vi "RingGetcam.VI"() -> ()   [LabVIEW 2014]
panel:
  in  "gain":bool
  in  "is FFT":bool
  out "FIFO overflow":bool
  in  "RingBufDepth":u32=100
  out "Signalverlaufgraph":u16[](graph)=[1244, 50394, 4112, 1253, 7937, 7970, 8022, 8007, 8036, 8064, 8081, 8047, 8038, 8131, 8189, 8160, 8237, 8217, 8253, 8234, 8286, 8282, 8333, 8330, 8377, 8354, 8432, 8412, 8472, 8454, 8502, 8506, 8551, 8555, 8618, 8587, 8654, 8622, 8678, 8676, 8705, 8728, 8760, 8721, 8806, 8782, 8832, 8816, 8851, 8867, 8922, 8915, 8965, 8956, 9002, 9006, 9029, 9038, 9114, 9050, 9101, 9142, 9164, 9171, 9207, 9200, 9261, 9214, 9288, 9285, 9307, 9310, 9364, 9322, 9368, 9404, 9444, 9436, 9485, 9469, 9497, 9508, 9551, 9587, 9619, 9562, 9655, 9637, 9680, 9710, 9733, 9765, 9805, 9794, 9828, 9847, 9877, 9892, 9929, 9953, 9984, 9976, 9964, 9951, 10046, 10054, 10122, 10146, 10138, 10167, 10220, 10223, 10221, 10209, 10262, 10275, 10311, 10336, 10323, 10329, 10396, 10389, 10431, 10441, 10499, 10494, 10530, 10518, 10556, 10581, 10574, 10588, 10671, 10647, 10718, 10692, 10736, 10737, 10788, 10775, 10817, 10833, 10901, 10910, 10918, 10969, 10979, 10881, 10950, 11009, 11047, 11098, 11107, 11147, 11163, 11162, 11227, 11210, 11262, 11276, 11309, 11281, 11376, 11389, 11416, 11363, 11442, 11440, 11474, 11467, 11544, 11546, 11578, 11588, 11602, 11640, 11674, 11702, 11752, 11734, 11773, 11843, 11822, 11884, 11908, 11894, 11970, 11945, 11982, 11998, 12097, 12075, 12138, 12095, 12193, 12189, 12212, 12229, 12270, 12291, 12316, 12311, 12403, 12336, 12398, 12436, 12438, 12466, 12529, 12485, 12567, 12474, 12519, 12605, 12658, 12644, 12686, 12689, 12758, 12769, 12800, 12781, 12848, 12835, 12800, 12899, 12934, 12922, 13024, 13029, 13054, 13029, 13052, 13056, 13115, 13124, 13177, 13229, 13227, 13212, 13273, 13273, 13364, 13298, 13388, 13369, 13398, 13353, 13433, 13426, 13527, 13481, 13577, 13517, 13573, 13564, 13572, 13572, 13630, 13597, 13724, 13640, 13703, 13749, 13749, 13746, 13754, 13800, 13805, 13805, 13882, 13865, 13820, 13884, 13937, 13915, 13930, 13952, 13982, 14022, 13992, 13984, 14010, 14082, 14053, 14123, 14116, 14130, 14144, 14159, 14198, 14243, 14153, 14275, 14233, 14252, 14251, 14226, 14320, 14319, 14348, 14346, 14307, 14362, 14346, 14373, 14418, 14408, 14450, 14449, 14438, 14444, 14449, 14483, 14516, 14485, 14475, 14519, 14516, 14561, 14568, 14495, 14574, 14601, 14562, 14574, 14687, 14606, 14639, 14616, 14580, 14563, 14564, 14492, 14612, 14666, 14666, 14627, 14605, 14651, 14562, 14602, 14586, 14639, 14612, 14622, 14632, 14624, 14627, 14670, 14637, 14638, 14652, 14612, 14667, 14577, 14675, 14615, 14603, 14613, 14608, 14582, 14645, 14567, 14603, 14581, 14593, 14515, 14581, 14588, 14590, 14566, 14567, 14586, 14557, 14493, 14517, 14501, 14490, 14520, 14513, 14498, 14502, 14469, 14489, 14444, 14453, 14452, 14458, 14453, 14463, 14453, 14448, 14427, 14459, 14382, 14402, 14352, 14369, 14426, 14350, 14315, 14341, 14328, 14321, 14268, 14298, 14298, 14318, 14275, 14286, 14227, 14279, 14249, 14266, 14253, 14225, 14186, 14236, 14203, 14197, 14200, 14185, 14168, 14209, 14119, 14127, 14163, 14152, 14114, 14117, 14079, 14082, 14116, 14086, 14056, 14040, 14058, 14033, 14039, 14048, 13952, 14027, 13906, 13953, 13961, 13966, 13982, 13947, 13921, 13874, 13930, 13882, 13880, 13830, 13856, 13830, 13817, 13770, 13812, 13775, 13798, 13791, 13744, 13744, 13687, 13664, 13686, 13638, 13662, 13637, 13598, 13593, 13587, 13548, 13559, 13505, 13541, 13509, 13489, 13458, 13461, 13421, 13418, 13400, 13398, 13277, 13368, 13269, 13313, 13273, 13235, 13281, 13233, 13186, 13193, 13117, 13169, 13073, 13102, 13049, 13071, 12996, 13021, 12938, 12993, 12920, 12972, 12920, 12918, 12865, 12878, 12764, 12758, 12725, 12717, 1287, 1294, 1292, 1293, 1295, 1295, 1299, 1297, 1296, 1293, 1292, 1291, 1292, 1290, 1287, 1287, 1290, 1282, 1281, 1278, 1281, 1276, 1279, 1283, 1272, 1273, 1276, 1280, 1273, 1271, 1273, 1273, 1271, 1274, 1272, 1266, 1267, 1259, 1267, 1264, 1259, 1265, 1258, 1260, 1261, 1261, 1262, 1261, 1262, 1259, 1257, 1254, 1260, 1258, 1257, 1258, 1259, 1254, 1251, 1253, 1254, 1254, 1250, 1252, 1251, 1256, 1254, 1254, 1253, 1248, 1247, 1255, 1247, 1250, 1248, 1243, 1252, 1251, 1255, 1252, 1249, 1251, 1249, 1249, 0, 0, 0, 0, 0, 0, 0, 0, 0, 0, 0, 0, 0, 0, 0, 0, 0, 0, 0, 0, 0, 0, 0, 0, 0, 0, 0, 0, 0, 0, 0, 0, 0, 0, 0, 0, 0, 0, 0, 0, 0, 0, 0, 0, 0, 0, 0, 0, 0, 0, 0, 0, 0, 0, 0, 0, 0, 0, 0, 0, 0, 0, 0, 0, 0, 0, 0, 0, 0, 0, 0, 0, 0, 0, 0, 0, 0, 0, 0, 0, 0, 0, 0, 0, 0, 0, 0, 0, 0, 0, 0, 0, 0, 0, 0, 0, 0, 0, 0, 0, 0, 0, 0, 0, 0, 0, 0, 0, 0, 0, 0, 0, 0, 0, 0, 0, 0, 0, 0, 0, 0, 0, 0, 0, 0, 0, 0, 0, 0, 0, 0, 0, 0, 0, 0, 0, 0, 0, 0, 0, 0, 0, 0, 0, 0, 0, 0, 0, 0, 0, 0, 0, 0, 0, 0, 0, 0, 0, 0, 0, 0, 0, 0, 0, 0, 0, 0, 0, 0, 0, 0, 0, 0, 0, 0, 0, 0, 0, 0, 0, 0, 0, 0, 0, 0, 0, 0, 0, 0, 0, 0, 0, 0, 0, 0, 0, 0, 0, 0, 0, 0, 0, 0, 0, 0, 0, 0, 0, 0, 0, 0, 0, 0, 0, 0, 0, 0, 0, 0, 0, 0, 0, 0, 0, 0, 0, 0, 0, 0, 0, 0, 0, 0, 0, 0, 0, 0, 0, 0, 0, 0, 0, 0, 0, 0, 0, 0, 0, 0, 0, 0, 0, 0, 0, 0, 0, 0, 0, 0, 0, 0, 0, 0, 0, 0, 0, 0, 0, 0, 0, 0, 0, 0, 0, 0, 0, 0, 0, 0, 0, 0, 0, 0, 0, 0, 0, 0, 0, 0, 0, 0, 0, 0, 0, 0, 0, 0, 0, 0, 0, 0, 0, 0, 0, 0, 0, 0, 0, 0, 0, 0, 0, 0, 0, 0, 0, 0, 0, 0, 0, 0, 0, 0, 0, 0, 0, 0, 0, 0, 0, 0, 0, 0, 0, 0, 0, 0, 0, 0, 0, 0, 0, 0, 0, 0, 0, 0, 0, 0, 0, 0, 0, 0, 0, 0, 0, 0, 0, 0, 0, 0, 0, 0, 0, 0, 0, 0, 0, 0, 0, 0, 0, 0, 0, 0, 0, 0, 0, 0, 0, 0, 0, 0, 0, 0, 0, 0, 0, 0, 0, 0, 0, 0, 0, 0, 0, 0, 0, 0, 0, 0, 0, 0, 0, 0, 0, 0, 0, 0, 0, 0, 0, 0, 0, 0, 0, 0, 0, 0, 0, 0, 0, 0, 0, 0, 0, 0, 0, 0, 0, 0, 0, 0, 0, 0, 0, 0, 0, 0, 0, 0, 0, 0, 0, 0, 0, 0, 0, 0, 0, 0, 0, 0, 0, 0, 0, 0, 0, 0, 0, 0, 0, 0, 0, 0, 0, 0, 0, 0, 0, 0, 0, 0, 0, 0, 0, 0, 0, 0, 0, 0, 0, 0, 0, 0, 0, 0, 0, 0, 0, 0, 0, 0, 0, 0, 0, 0, 0, 0, 0, 0, 0, 0, 0, 0, 0, 0, 0, 0, 0, 0, 0, 0, 0, 0, 0, 0, 0, 0, 0, 0, 0, 0, 0, 0, 0, 0, 0, 0, 0, 0, 0, 0, 0, 0, 0, 0, 0, 0, 0, 0, 0, 0, 0, 0, 0, 0, 0, 0, 0, 0, 0, 0, 0, 0, 0, 0, 0, 0, 0, 0, 0, 0, 0, 0, 0, 0, 0, 0, 0, 0, 0, 0, 0, 0, 0, 0, 0, 0, 0, 0, 0, 0, 0, 0, 0, 0, 0, 0, 0, 0, 0, 0, 0, 0, 0, 0, 0, 0, 0]
  in  "Trigger":bool
  in  "Stop":bool
  in  "ClrReads":u32=4
  in  "exposuretime":dbl=1.0 format="%.2f"
  # "Start with run"
  # "be shure to use lower stop button or ESC to quit - or thread will keep on going!"
  # "in ms"
  # "ext"
  # "int"
  # "IR"
  # "lo"
  # "hi"
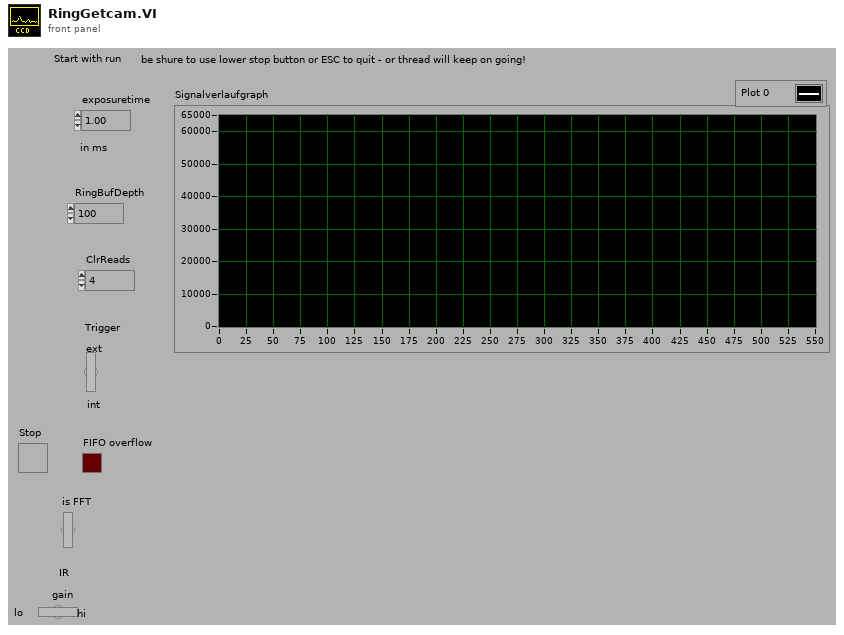
[diagram p1: front panel]
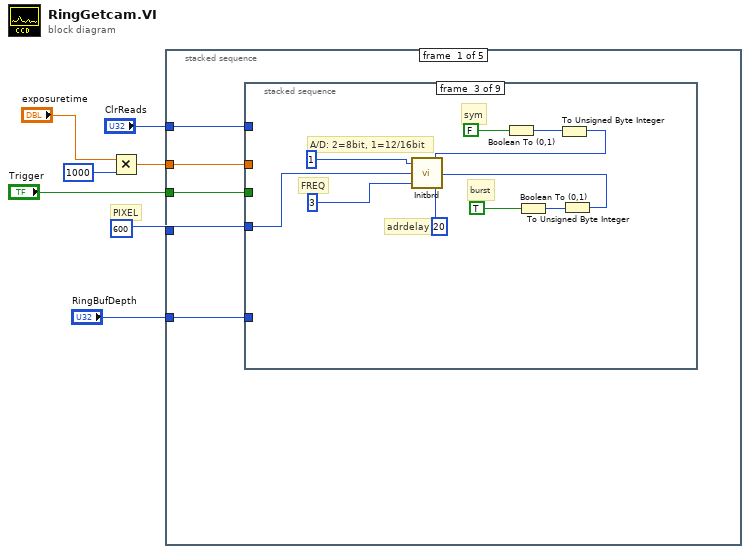
[diagram p0: block diagram]
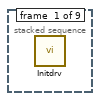
[diagram p2: hidden frame]
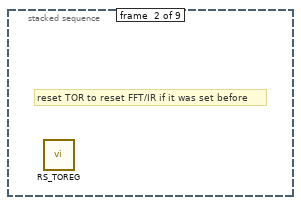
[diagram p3: hidden frame]
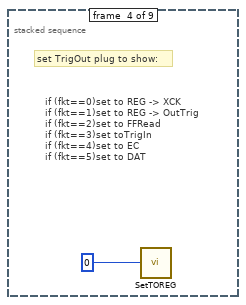
[diagram p4: hidden frame]
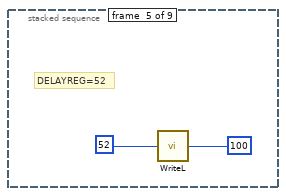
[diagram p5: hidden frame]
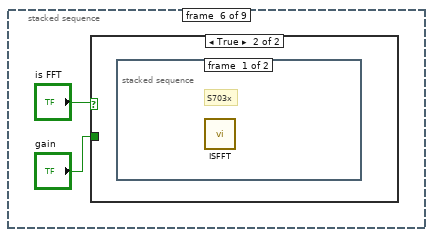
[diagram p6: hidden frame]
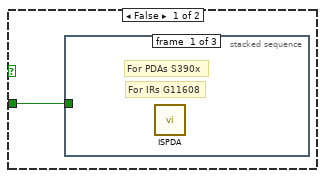
[diagram p7: hidden frame]
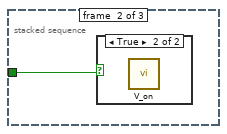
[diagram p8: hidden frame]
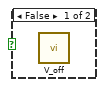
[diagram p9: hidden frame]
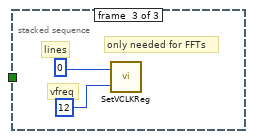
[diagram p10: hidden frame]
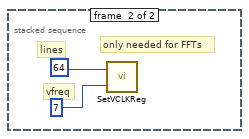
[diagram p11: hidden frame]
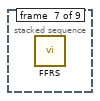
[diagram p12: hidden frame]
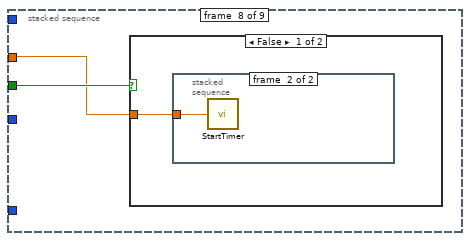
[diagram p13: hidden frame]
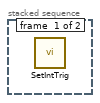
[diagram p14: hidden frame]
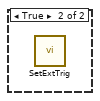
[diagram p15: hidden frame]
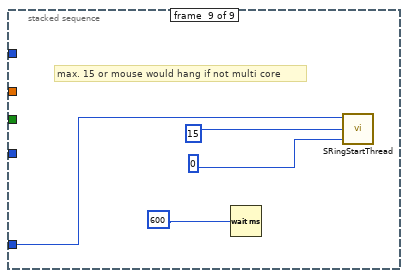
[diagram p16: hidden frame]
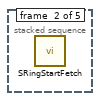
[diagram p17: hidden frame]
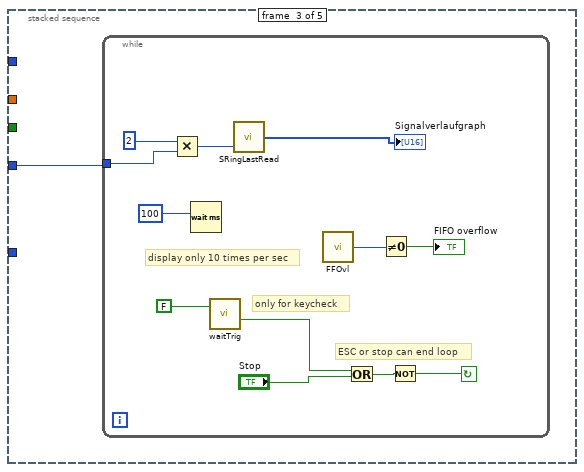
[diagram p18: hidden frame]
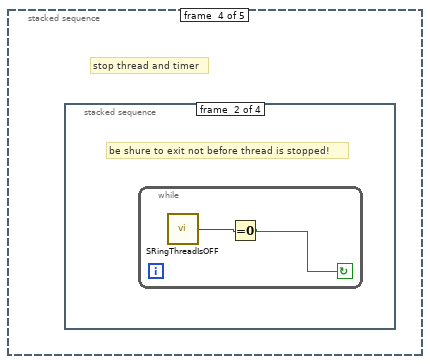
[diagram p19: hidden frame]
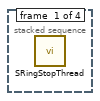
[diagram p20: hidden frame]
diagram:
  # "PIXEL"
  n1 = Multiply(x="exposuretime", y=1000) -> (x*y=w3:dbl)
  n2 = stacked-sequence {
    tunnel: w3 -> [w11 _ _ _ _]
    tunnel: u32 600 -> [w12 _ w42 _ _]
    tunnel: "ClrReads" -> [w10 _ _ _ _]
    tunnel: "Trigger" -> [w9 _ _ _ _]
    tunnel: "RingBufDepth" -> [w8 _ _ _ _]
    frame #0 {
      n3 = stacked-sequence {
        tunnel: w12 -> [_ _ w21 _ _ _ _ _ _]
        tunnel: w11 -> [_ _ _ _ _ _ _ w34 _]
        tunnel: w10 -> [_ _ _ _ _ _ _ _ _]
        tunnel: w9 -> [_ _ _ _ _ _ _ w35 _]
        tunnel: w8 -> [_ _ _ _ _ _ _ _ w38]
        frame #0 {
          n4 = call "Initdrv.vi"() -> ()  [unwired: 1 in]
        }
        frame #1 {
          # "reset TOR to reset FFT/IR if it was set before"
          n5 = call "RS_TOREG.vi"() -> ()  [unwired: 1 in]
        }
        frame #2 {
          # "adrdelay"
          # "FREQ"
          # "A/D: 2=8bit, 1=12/16bit"
          # "burst"
          # "sym"
          n6 = Boolean To (0,1)(Boolean=FALSE) -> (0, 1=w15:i16)
          n7 = Boolean To (0,1)(Boolean=TRUE) -> (0, 1=w14:i16)
          n8 = To Unsigned Byte Integer(number=w15) -> (unsigned 8bit integer=w16:u8)
          n9 = To Unsigned Byte Integer(number=w14) -> (unsigned 8bit integer=w13:u8)
          n10 = call "Initbrd.vi"("AdrDelay"=u32 20, "burst"=w13, "sym"=w16, "waits"=u32 3, "pixel"=w21, "flag816"=u32 1) -> ()
        }
        frame #3 {
          # "set TrigOut plug to show:"
          # "if (fkt==0)set to REG -> XCK\nif (fkt==1)set to REG -> OutTrig\nif (fkt==2)set to FFRead\nif (fkt==3)set toTrigIn\nif (fkt==4)set to EC\nif (fkt==5)set to DAT"
          n11 = call "SetTOREG.vi"("fkt"=u8 0) -> ()
        }
        frame #4 {
          # "DELAYREG=52"
          n12 = call "WriteL.vi"("val"=u32 100, "offset"=u32 52) -> ()
        }
        frame #5 {
          n13 = case shown="True" "is FFT" {
            tunnel: "gain" -> [w28 _]
            frame False {
              n14 = stacked-sequence {
                tunnel: w28 -> [_ w29 _]
                frame #0 {
                  # "For IRs G11608"
                  # "For PDAs S390x"
                  n15 = call "ISPDA.vi"() -> ()  [unwired: 1 in]
                }
                frame #1 {
                  n16 = case shown="True" w29 {
                    frame False {
                      n17 = call "V_off.vi"() -> ()  [unwired: 1 in]
                    }
                    frame True {
                      n18 = call "V_on.vi"() -> ()  [unwired: 1 in]
                    }
                  }
                }
                frame #2 {
                  # "only needed for FFTs"
                  # "vfreq"
                  # "lines"
                  n19 = call "SetVCLKReg.vi"("vfreq"=u8 12, "lines"=u32 0) -> ()  [unwired: 1 in]
                }
              }
            }
            frame True {
              n20 = stacked-sequence {
                frame #0 {
                  # "S703x"
                  n21 = call "ISFFT.vi"() -> ()  [unwired: 1 in]
                }
                frame #1 {
                  # "only needed for FFTs"
                  # "vfreq"
                  # "lines"
                  n22 = call "SetVCLKReg.vi"("vfreq"=7, "lines"=64) -> ()  [unwired: 1 in]
                }
              }
            }
          }
        }
        frame #6 {
          n23 = call "FFRS.VI"() -> ()  [unwired: 1 in]
        }
        frame #7 {
          n24 = case shown="False" w35 {
            tunnel: w34 -> [w36 _]
            frame False {
              n25 = stacked-sequence {
                tunnel: w36 -> [_ w37]
                frame #0 {
                  n26 = call "SetIntTrig.vi"() -> ()  [unwired: 1 in]
                }
                frame #1 {
                  n27 = call "StartTimer.vi"("exposure time"=w37) -> ()  [unwired: 1 in]
                }
              }
            }
            frame True {
              n28 = call "SetExtTrig.vi"() -> ()  [unwired: 1 in]
            }
          }
        }
        frame #8 {
          # "max. 15 or mouse would hang if not multi core"
          n29 = Wait (ms)(milliseconds to wait=u32 600) -> ()  [unwired: 1 out]
          n30 = call "SRingStartThread.vi"("releasems"=i16 0, "threadp"=u32 15, "ringdepth"=w38) -> ()  [unwired: 1 in]
        }
      }
    }
    frame #1 {
      n31 = call "SRingStartFetch.vi"() -> ()  [unwired: 2 in]
    }
    frame #2 {
      n32 = while {
        tunnel: w42 -> [w52]
        stop <- w54 continue-if-true
        # "only for keycheck"
        # "ESC or stop can end loop"
        # "display only 10 times per sec"
        n33 = Multiply(x=2, y=w52) -> (x*y=w51:u32)
        n34 = Wait (ms)(milliseconds to wait=100) -> ()  [unwired: 1 out]
        n35 = call "waitTrig.vi"("Trigger\nextern"=FALSE) -> ("ESCKey"=w47:bool)  [unwired: 1 in, 1 out]
        n36 = call "SRingLastRead.vi"("pixel"=w51) -> ("Data Values"=→"Signalverlaufgraph":u16[])  [unwired: 2 in]
        n37 = call "FFOvl.vi"() -> ("FFOvl"=w45:u8)  [unwired: 1 in]
        n38 = Or(x=w47, y="Stop") -> (x .or. y?=w46:bool)
        n39 = Not Equal To 0?(x=w45) -> (x != 0?=→"FIFO overflow":bool)
        n40 = Not(x=w46) -> (.not. x?=w54:bool)
      }
    }
    frame #3 {
      # "stop thread and timer"
      n41 = stacked-sequence {
        frame #0 {
          n42 = call "SRingStopThread.vi"() -> ()  [unwired: 4 in]
        }
        frame #1 {
          # "be shure to exit not before thread is stopped!"
          n43 = while {
            stop <- w55 continue-if-true
            n44 = call "SRingThreadIsOFF.vi"() -> ("ThreadIsOFF"=w56:u8)  [unwired: 1 in]
            n45 = Equal To 0?(x=w56) -> (x = 0?=w55:bool)
          }
        }
        frame #2 {
          n46 = call "FFStopTimer.vi"() -> ()  [unwired: 1 in]
        }
        frame #3 {
          # "stops ext trigger from running"
          n47 = call "SetIntTrig.vi"() -> ()  [unwired: 1 in]
        }
      }
    }
    frame #4 {
      n48 = call "Exit.vi"() -> ()  [unwired: 1 in]
    }
  }
